vi "WriteToBuffers.vi"(0 "Buffers in":T1={"Channels"=[], "PosttriggerBuffer"=refnum, "PretriggerBuffer"=refnum, "BlockSizePerChannel"=0, " logging semaphore"=refnum, "Log refnum"=refnum, "snapshotBuffer"=refnum, "logDirectory"=path "", "logPrefix"="", "decimation factor"=1, "max files"=0, "SampleRate"=0.0}, 5 "Data":sgl[](array[numeric]), 11 "error in (no error)":errorcluster) -> (4 "Buffers out":T1={"Channels"=[], "PosttriggerBuffer"=refnum, "PretriggerBuffer"=refnum, "BlockSizePerChannel"=0, " logging semaphore"=refnum, "Log refnum"=refnum, "snapshotBuffer"=refnum, "logDirectory"=path "", "logPrefix"="", "decimation factor"=1, "max files"=0, "SampleRate"=0.0}, 15 "error out":errorcluster)   [LabVIEW 2017, in "BufferLogging.lvlib"]
doc: "Write to the pretrigger and posttrigger buffers."
uses:
  BufferLogging.lvlib
  Buffers.ctl
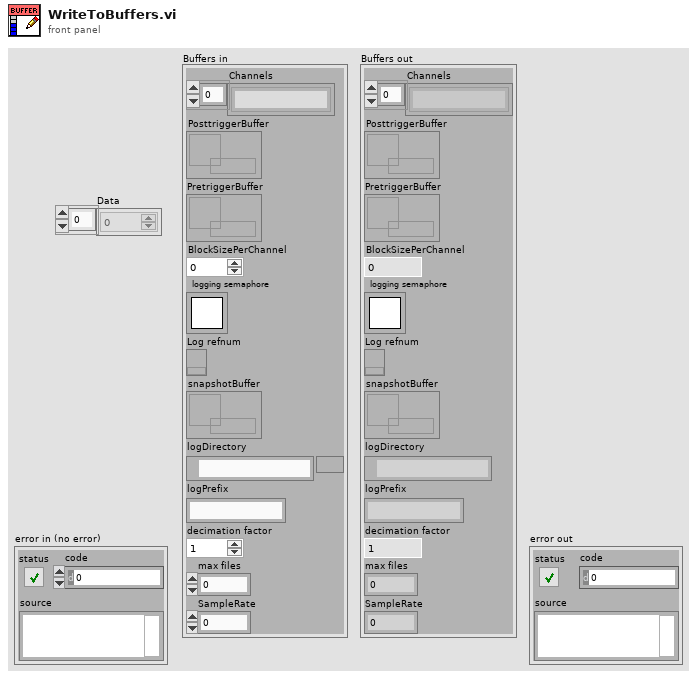
[diagram p1: front panel]
types:
  T1 = typedef "BufferLogging.lvlib/Buffers.ctl" = cluster{"Channels":string[], "PosttriggerBuffer":refnum<queue>, "PretriggerBuffer":refnum<queue>, "BlockSizePerChannel":i32, " logging semaphore":T2, "Log refnum":refnum<k34>, "snapshotBuffer":refnum<data-value>, "logDirectory":path, "logPrefix":string, "decimation factor":i32, "max files":i32, "SampleRate":dbl}
  T2 = typedef "Semaphore RefNum" = refnum<k1>
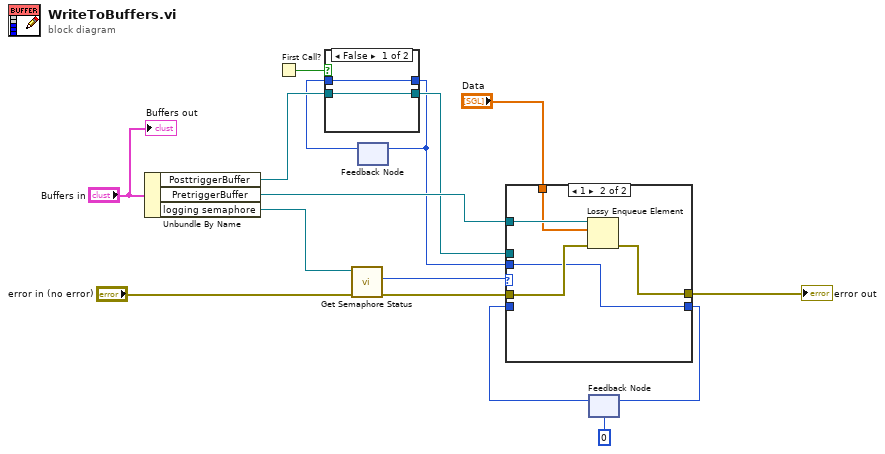
[diagram p0: block diagram]
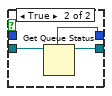
[diagram p2: hidden frame]
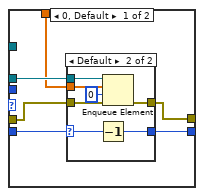
[diagram p3: hidden frame]
diagram:
  n1 = Unbundle By Name("Buffers in") -> ("PosttriggerBuffer"=w8:refnum<queue>, "PretriggerBuffer"=w6:refnum<queue>, "logging semaphore"=w12:T2)
  n2 = First Call?() -> (First Call?: T/F=w9:bool)
  n3 = call <vilib>:"Get Semaphore Status.vi"("error in (no error)"="error in (no error)", "semaphore"=w12) -> ("error out"=w10:errorcluster, "# available"=w16:i32)  [unwired: 4 in, 4 out]
  n4 = feedback #1() -> (w7:i32)  [unwired: 1 in]
  n5 = case shown="False" w9 {
    tunnel: w8 -> [w18 w21]
    tunnel: [w18 w20] -> w5
    tunnel: [w17 w19] -> w3
    tunnel: w7 -> [w17 _]
    frame False {
    }
    frame True {
      n6 = Get Queue Status(queue=w21) -> (queue out=w20:refnum<queue>, max queue size=w19:i32)  [unwired: 2 in, 6 out]
    }
  }
  n7 = feedback-in #1(w3) -> ()
  n8 = feedback #2(0 ("max queue size")) -> (w1:i32)
  n9 = case shown="1" w16 {
    tunnel: w6 -> [_ w41]
    tunnel: "Data" -> [w25 w40]
    tunnel: w10 -> [w26 w39]
    tunnel: [w24 w38] -> w15
    tunnel: w5 -> [w27 _]
    tunnel: w3 -> [_ w37]
    tunnel: [w23 w37] -> w2
    tunnel: w1 -> [w22 _]
    frame 0, Default {
      n10 = case shown="Default" w22 {
        selector: w22 -> [w29 w31]
        tunnel: w27 -> [_ w36]
        tunnel: w26 -> [w28 w35]
        tunnel: w25 -> [_ w34]
        tunnel: [w29 w32] -> w23
        tunnel: [w28 w30] -> w24
        frame 0 {
        }
        frame Default {
          n11 = Decrement(x=w31) -> (x-1=w32:i32)
          n12 = Enqueue Element(queue=w36, element=w34, timeout in ms (-1)=0, error in (no error)=w35) -> (error out=w30:errorcluster)  [unwired: 2 out]
        }
      }
    }
    frame 1 {
      n13 = Lossy Enqueue Element(queue=w41, element=w40, error in (no error)=w39) -> (error out=w38:errorcluster)  [unwired: 3 out]
    }
  }
  "error out" <- w15
  n14 = feedback-in #2(w2) -> ()
  "Buffers out" <- "Buffers in"
